vi "blueScreenTest.vi"() -> ()   [LabVIEW 2009, in "run.lvlib"]
uses:
  run.lvlib
  HWController/Network Controllers/NetworkCamera/NetworkCamera.lvclass
  Tools/Filing/FileSystem/FileSystem.lvclass
  Tools/CameraSettings/CamaraSettings.lvclass
  Tools/Filing/FileNeologist/FileNeologist.lvclass
panel:
  out "stopped?":bool
  in  "stop":bool
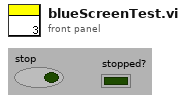
[diagram p1: front panel]
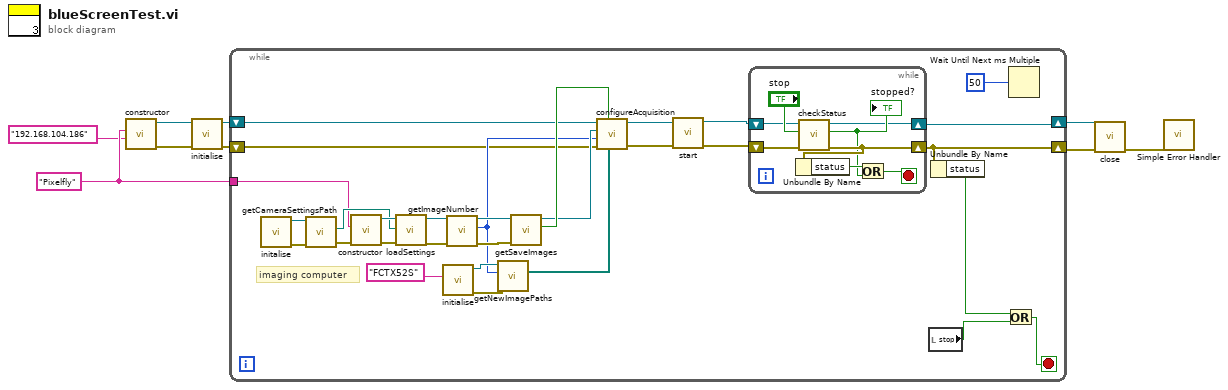
[diagram p0: block diagram]
diagram:
  w5 = "Pixelfly"
  n1 = call "constructor.vi"("machine name"="192.168.104.186", "Camera"=w5) -> ("error out"=w6:errorcluster, "NetworkCamera out"=w7:refnum<class "NetworkCamera.lvclass">)  [unwired: 8 in]
  n2 = call-dynamic "initialise.vi"("error in (no error)"=w6, "NetworkCamera in"=w7) -> ("error out"=w8:errorcluster, "NetworkCamera out"=w9:refnum<class "NetworkCamera.lvclass">)  [unwired: 8 in]
  n3 = while {
    tunnel: w5 -> [w16]
    shift-right: [w11] -> w2
    shift-left: w8 -> [w17]
    shift-right: [w10] -> w3
    shift-left: w9 -> [w18]
    stop <- w15 stop-if-true
    # "imaging computer"
    n4 = call "initalise.vi"() -> ("error out"=w38:errorcluster, "FileSystem out"=w39:refnum<class "FileSystem.lvclass">)  [unwired: 10 in]
    n5 = call-dynamic "getCameraSettingsPath.vi"("error in (no error)"=w38, "FileSystem.lvclass in"=w39) -> ("error out"=w36:errorcluster, "CameraSettingsPath"=w35:path)  [unwired: 7 in, 1 out]
    n6 = call "constructor.vi"("error in (no error)"=w36, "camera settings"=w16) -> ("error out"=w34:errorcluster, "CamaraSettings out"=w37:refnum<class "CamaraSettings.lvclass">)  [unwired: 8 in]
    n7 = call-dynamic "loadSettings.vi"("error in (no error)"=w34, "Path"=w35, "CamaraSettings in"=w37) -> ("error out"=w32:errorcluster, "CamaraSettings out"=w33:refnum<class "CamaraSettings.lvclass">)  [unwired: 7 in]
    n8 = call "initialise.vi"("computer name"="FCTX52S") -> ("error out"=w27:errorcluster, "FileNeologist out"=w28:refnum<class "FileNeologist.lvclass">)  [unwired: 9 in]
    n9 = call-dynamic "getImageNumber.vi"("error in (no error)"=w32, "CamaraSettings in"=w33) -> ("error out"=w30:errorcluster, "image number"=w24:i32, "CamaraSettings out"=w31:refnum<class "CamaraSettings.lvclass">)  [unwired: 7 in]
    n10 = call "getNewImagePaths.vi"("error in (no error)"=w27, "numberOfImages"=w24, "FileNeologist in"=w28) -> ("Paths"=w23:path[])  [unwired: 6 in, 2 out]
    n11 = call "getSaveImages.vi"("error in (no error)"=w30, "CamaraSettings in"=w31) -> ("saveImages"=w29:bool, "CamaraSettings out"=w25:refnum<class "CamaraSettings.lvclass">)  [unwired: 7 in, 1 out]
    n12 = call-dynamic "configureAcquisition.vi"("imagePaths"=w23, "saveImages?"=w29, "error in (no error)"=w17, "number of Images"=w24, "CamaraSettings"=w25, "NetworkCamera in"=w18) -> ("error out"=w21:errorcluster, "NetworkCamera out"=w22:refnum<class "NetworkCamera.lvclass">)  [unwired: 4 in]
    n13 = call-dynamic "start.vi"("error in (no error)"=w21, "NetworkCamera in"=w22) -> ("error out"=w19:errorcluster, "NetworkCamera out"=w20:refnum<class "NetworkCamera.lvclass">)  [unwired: 8 in]
    n14 = while {
      shift-right: [w44] -> w11
      shift-left: w19 -> [w46]
      shift-right: [w40] -> w10
      shift-left: w20 -> [w41]
      stop <- w42 stop-if-true
      n15 = call-dynamic "checkStatus.vi"("error in (no error)"=w46, "stop"="stop", "NetworkCamera in"=w41) -> ("error out"=w44:errorcluster, "stopped?"=w43:bool, "NetworkCamera out"=w40:refnum<class "NetworkCamera.lvclass">)  [unwired: 6 in]
      "stopped?" <- w43
      n16 = Unbundle By Name(w44) -> ("status"=w45:bool)
      n17 = Or(x=w45, y=w43) -> (x .or. y?=w42:bool)
    }
    n18 = local read "stop"() -> (w13:bool)
    n19 = Unbundle By Name(w11) -> ("status"=w14:bool)
    n20 = Or(x=w14, y=w13) -> (x .or. y?=w15:bool)
    n21 = Wait Until Next ms Multiple(millisecond multiple=50) -> ()  [unwired: 1 out]
  }
  n22 = call-dynamic "close.vi"("error in (no error)"=w2, "NetworkCamera in"=w3) -> ("error out"=w1:errorcluster)  [unwired: 9 in]
  n23 = call <vilib>:"Simple Error Handler.vi"("error in (no error)"=w1) -> ()  [unwired: 4 in, 5 out]
